vi "Write All Child Attributes.vi"(10 "All Child Attributes":T1, 11 "Core Actor in":refnum<class "Core Actor.lvclass">) -> (3 "Core Actor out":refnum<class "Core Actor.lvclass">)   [LabVIEW 2025, in "jettl.lvlib" / "Base Actor.lvlib" / "Core Actor.lvclass"]
uses:
  Core Actor.lvclass
  All Child Attributes.ctl
  Attributes/Attributes.lvclass
  Core Actor.lvclass/Core Actor.ctl
  jettl.lvlib
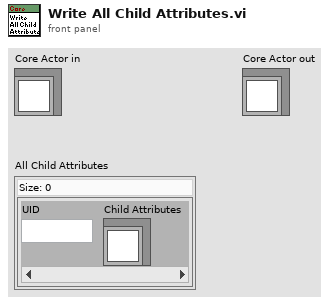
[diagram p1: front panel]
types:
  T1 = typedef "jettl.lvlib/All Child Attributes.ctl" = map{string, refnum<class "Attributes.lvclass">}
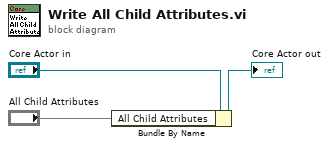
[diagram p0: block diagram]
diagram:
  n1 = Bundle By Name(cluster="Core Actor in", "All Child Attributes"="All Child Attributes") -> (→"Core Actor out":refnum<class "Core Actor.lvclass">)
